vi "Remove 2D Array Global Outliers (SGL).vi"(8 "Error In":errorcluster, 10 "Percentile (0-100, Default: ignore)":dbl min=0.0 max=100.0, 11 "2D Array in":sgl[][](array[numeric])) -> (0 "Error Out":errorcluster, 2 "# Modified Values":i32, 3 "2D Array out":sgl[][](array[numeric]))   [LabVIEW 2021, in "Arrays.lvlib"]
uses:
  Arrays.lvlib
  b07ea3fb-22b5-4eaf-9979-b69b03fc0317.vi
  b07ea3fb-22b5-4eaf-9979-b69b03fc0317.vi/3663a709-d1bc-4b7c-975a-3a90df5366f4.vi
  Utilities/Utilities.lvlib
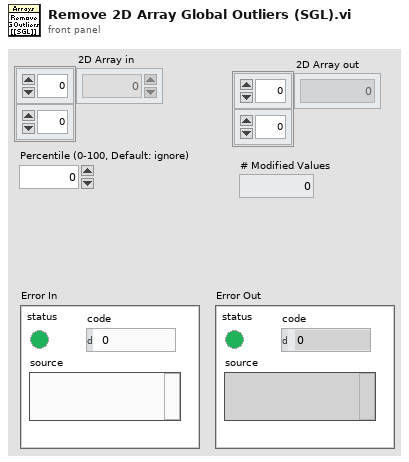
[diagram p1: front panel]
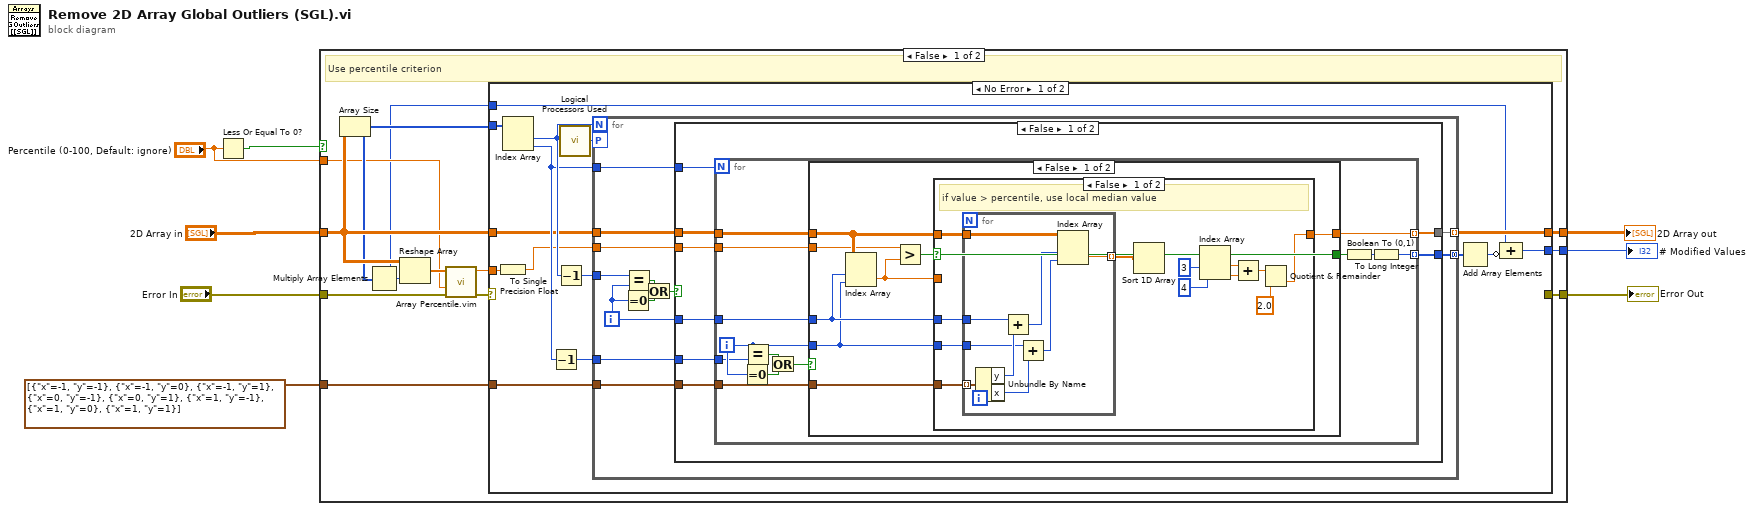
[diagram p0: block diagram]
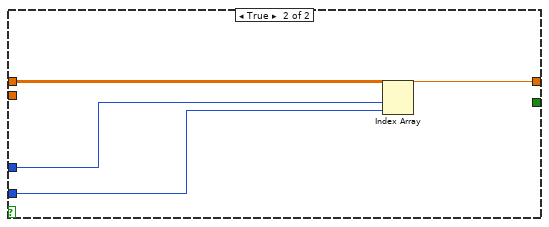
[diagram p3: hidden frame]
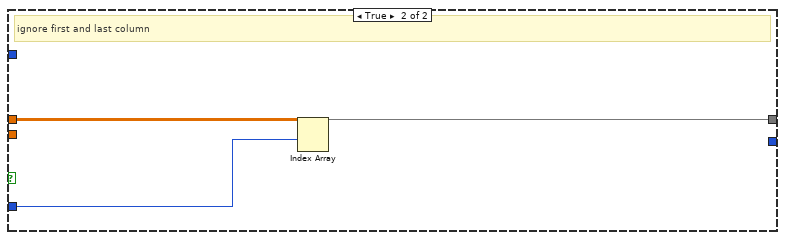
[diagram p4: hidden frame]
diagram:
  n1 = Less Or Equal To 0?(x="Percentile (0-100, Default: ignore)") -> (x <= 0?=w8:bool)
  n2 = case shown="False" w8 {
    tunnel: cluster{"x":i32, "y":i32}[] [{"x"=-1, "y"=-1}, {"x"=-1, "y"=0}, {"x"=-1, "y"=1}, {"x"=0, "y"=-1}, {"x"=0, "y"=1}, {"x"=1, "y"=-1}, {"x"=1, "y"=0}, {"x"=1, "y"=1}] -> [w20 _]
    tunnel: [w19 w110] -> w2
    tunnel: "2D Array in" -> [w17 w110]
    tunnel: "Error In" -> [w15 w109]
    tunnel: [w13 w109] -> w3
    tunnel: "Percentile (0-100, Default: ignore)" -> [w11 _]
    tunnel: [w10 _] -> w1
    frame False {
      # "Use percentile criterion"
      n3 = Array Size(array=w17) -> (size(s)=w16:i32[])
      n4 = Multiply Array Elements(1:w16) -> (0:w9:i32)
      n5 = Reshape Array(w17, w9) -> (w18:sgl[])
      n6 = call "Array Percentile.vim"("Error In"=w15, "Percentile (0-100)"=w11, "Array"=w18) -> ("Error Out"=w14:errorcluster, "Percentile Value"=w12:sgl)  [unwired: 7 in]
      n7 = case shown="No Error" w14 {
        selector: w14 -> [_ w107]
        tunnel: w20 -> [w35 _]
        tunnel: [w34 w108] -> w19
        tunnel: w17 -> [w29 w108]
        tunnel: w16 -> [w28 _]
        tunnel: [_ w107] -> w13
        tunnel: w12 -> [w27 _]
        tunnel: [w22 _] -> w10
        tunnel: w9 -> [w21 _]
        frame No Error {
          n8 = To Single Precision Float(number=w27) -> (single precision float=w26:sgl)
          n9 = Index Array(array=w28) -> (element #1=w33:i32, element #2=w31:i32)  [unwired: 2 in]
          n10 = Decrement(x=w31) -> (x-1=w30:i32)
          n11 = Decrement(x=w33) -> (x-1=w32:i32)
          n12 = call "Logical Processors Used.vi"() -> ("# Logical Processor Used"=w25:i32)  [unwired: 6 in]
          n13 = for {
            N: w33 -> [_]
            tunnel: w29 -> [w47]
            tunnel: w35 -> [w46]
            tunnel: [w45] -> w34 mode=indexing
            tunnel: w31 -> [w44]
            tunnel: w32 -> [w42]
            tunnel: w30 -> [w38]
            tunnel: w26 -> [w37]
            workers-P: w25 -> [_]
            tunnel: [w36] -> w24 mode=concatenating
            i -> [w43]
            n14 = Equal To 0?(x=w43) -> (x = 0?=w40:bool)
            n15 = Equal?(x=w42, y=w43) -> (x = y?=w41:bool)
            n16 = Or(x=w41, y=w40) -> (x .or. y?=w39:bool)
            n17 = case shown="False" w39 {
              tunnel: w47 -> [w55 w106]
              tunnel: w46 -> [w54 _]
              tunnel: [w53 w104] -> w45
              tunnel: w44 -> [w52 _]
              tunnel: w43 -> [w50 w105]
              tunnel: w38 -> [w51 _]
              tunnel: w37 -> [w49 _]
              tunnel: [w48 _] -> w36
              frame False {
                n18 = for {
                  N: w52 -> [_]
                  tunnel: w50 -> [w66]
                  tunnel: w55 -> [w67]
                  tunnel: w54 -> [w68]
                  tunnel: [w65] -> w53 mode=indexing
                  tunnel: w51 -> [w61]
                  tunnel: w49 -> [w59]
                  tunnel: [w56] -> w48 mode=indexing
                  i -> [w62]
                  n19 = Equal To 0?(x=w62) -> (x = 0?=w64:bool)
                  n20 = Equal?(x=w62, y=w61) -> (x = y?=w63:bool)
                  n21 = Or(x=w63, y=w64) -> (x .or. y?=w60:bool)
                  n22 = case shown="False" w60 {
                    tunnel: w68 -> [w76 _]
                    tunnel: w67 -> [w75 w103]
                    tunnel: w66 -> [w74 w102]
                    tunnel: [w71 w100] -> w65
                    tunnel: w62 -> [w73 w101]
                    tunnel: w59 -> [w72 _]
                    tunnel: [w69 _] -> w58
                    frame False {
                      n23 = Index Array(array=w75, index (row)=w74, index (col)=w73) -> (element=w70:sgl)
                      n24 = Greater?(x=w72, y=w70) -> (0:w69:bool)
                      n25 = case shown="False" w69 {
                        tunnel: w76 -> [w89 _]
                        tunnel: w75 -> [w82 _]
                        tunnel: w74 -> [w81 _]
                        tunnel: w73 -> [w80 _]
                        tunnel: [w79 w99] -> w71
                        tunnel: w70 -> [_ w99]
                        frame False {
                          # "if value > percentile, use local median value"
                          n26 = for {
                            tunnel: w82 -> [w93]
                            tunnel: w89 -> [w98] mode=indexing
                            tunnel: w81 -> [w97]
                            tunnel: w80 -> [w95]
                            tunnel: [w90] -> w78 mode=indexing
                            n27 = Unbundle By Name(w98) -> ("y"=w96:i32, "x"=w94:i32)
                            n28 = Add(x=w97, y=w96) -> (x+y=w92:i32)
                            n29 = Add(x=w95, y=w94) -> (x+y=w91:i32)
                            n30 = Index Array(array=w93, index (row)=w92, index (col)=w91) -> (element=w90:sgl)
                          }
                          n31 = Sort 1D Array(array=w78) -> (sorted array=w77:sgl[])
                          n32 = Index Array(array=w77, index #1=3 ("index"), index #2=4 ("index")) -> (element #1=w86:sgl, element #2=w85:sgl)
                          n33 = Add(x=w86, y=w85) -> (x+y=w84:sgl)
                          n34 = Quotient & Remainder(x=w84, y=sgl 2.0) -> (floor(x/y)=w79:sgl)  [unwired: 1 out]
                        }
                        frame True {
                          # "if value < percentile value, keep it"
                        }
                      }
                    }
                    frame True {
                      # "ignore first and last row"
                      n35 = Index Array(array=w103, index (row)=w102, index (col)=w101) -> (element=w100:sgl)
                    }
                  }
                  n36 = Boolean To (0,1)(Boolean=w58) -> (0, 1=w57:i16)
                  n37 = To Long Integer(number=w57) -> (32bit integer=w56:i32)
                }
              }
              frame True {
                # "ignore first and last column"
                n38 = Index Array(array=w106, index (row)=w105) -> (element=w104:sgl[])  [unwired: 1 in]
              }
            }
          }
          n39 = Add Array Elements(numeric array=w24) -> (sum=w23:i32)
          n40 = Compound Arithmetic op=ADD(w21, invert w23) -> (w22:i32)
        }
        frame Error {
        }
      }
    }
    frame True {
      # "do nothing"
    }
  }
  "Error Out" <- w3
  "2D Array out" <- w2
  "# Modified Values" <- w1
